vi "Increment File Counter.vi"(8 "error in (no error)":errorcluster, 10 "File Path":path, 11 "Text File Sink in":refnum<class "Text File Sink.lvclass">) -> (0 "error out":errorcluster, 2 "File Path out":path, 3 "Text File Sink out":refnum<class "Text File Sink.lvclass">)   [LabVIEW 2016, in "Stream Log.lvlib" / "Text File Sink.lvclass"]
uses:
  <userlib>/Composed Systems/Stream/Log/Text File Sink/Text File Sink.lvclass
  <userlib>/Composed Systems/Stream/Log/Text File Sink/Text File Sink.lvclass/Text File Sink.ctl
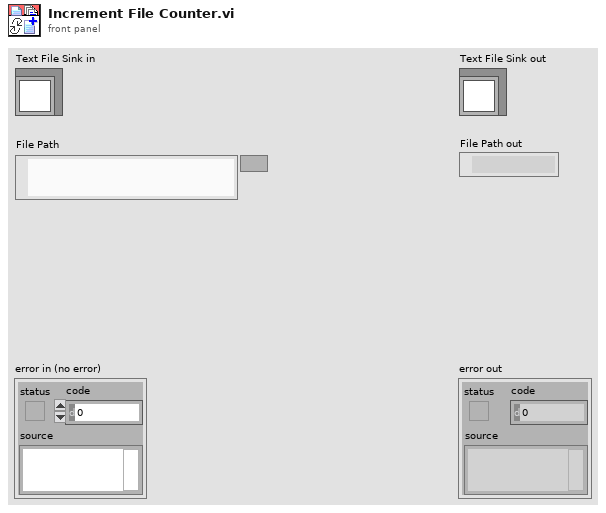
[diagram p1: front panel]
types:
  T1 = typedef "LVDateTimeRec.ctl" = cluster{"fractional second":dbl, "second":i32, "minute":i32, "hour":i32, "day of month":i32, "month":i32, "year":i32, "day of week":i32, "day of year":i32, "DST":i32}
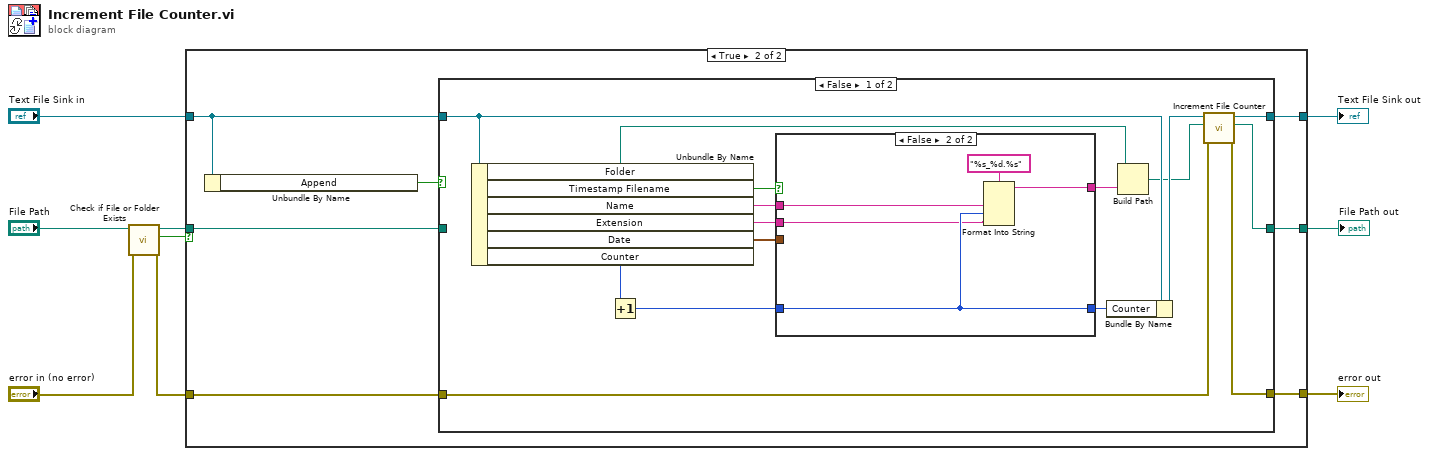
[diagram p0: block diagram]
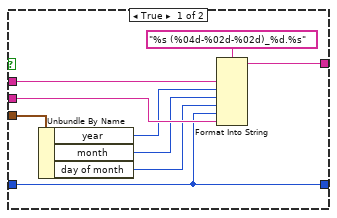
[diagram p3: hidden frame]
diagram:
  n1 = call <vilib>:"Check if File or Folder Exists.vi"("error in (no error)"="error in (no error)", "path"="File Path") -> ("error out"=w2:errorcluster, "file or folder exists?"=w9:bool, "dup path"=w8:path)  [unwired: 7 out]
  n2 = case shown="True" w9 {
    tunnel: w8 -> [w12 w16]
    tunnel: [w12 w17] -> w3
    tunnel: [w11 w15] -> w6
    tunnel: "Text File Sink in" -> [w11 w19]
    tunnel: [w10 w13] -> w1
    tunnel: w2 -> [w10 w14]
    frame False {
    }
    frame True {
      n3 = Unbundle By Name(w19) -> ("Append"=w18:bool)
      n4 = case shown="False" w18 {
        tunnel: [w26 w52] -> w15
        tunnel: w19 -> [w30 w52]
        tunnel: [w25 w51] -> w17
        tunnel: w16 -> [_ w51]
        tunnel: w14 -> [w24 w50]
        tunnel: [w23 w50] -> w13
        frame False {
          n5 = Unbundle By Name(w30) -> ("Folder"=w31:path, "Timestamp Filename"=w20:bool, "Name"=w35:string, "Extension"=w34:string, "Date"=w33:T1, "Counter"=w28:u16)
          n6 = Increment(x=w28) -> (x+1=w29:u16)
          n7 = case shown="False" w20 {
            tunnel: w35 -> [w43 w48]
            tunnel: w34 -> [w42 w45]
            tunnel: w33 -> [w41 _]
            tunnel: [w37 w47] -> w32
            tunnel: w29 -> [w36 w46]
            tunnel: [w36 w46] -> w21
            frame True {
              n8 = Unbundle By Name(w41) -> ("year"=w40:i32, "month"=w39:i32, "day of month"=w38:i32)
              n9 = Format Into String(format string="%s (%04d-%02d-%02d)_%d.%s", w43, w40, w39, w38, w36, w42) -> (resulting string=w37:string)  [unwired: 2 in, 1 out]
            }
            frame False {
              n10 = Format Into String(format string="%s_%d.%s", w48, w46, w45) -> (resulting string=w47:string)  [unwired: 2 in, 1 out]
            }
          }
          n11 = Bundle By Name(cluster=w30, "Counter"=w21) -> (w27:refnum<class "Text File Sink.lvclass">)
          n12 = Build Path(base path=w31, name or relative path=w32) -> (appended path=w22:path)
          n13 = call <userlib>:"Increment File Counter.vi"("error in (no error)"=w24, "File Path"=w22, "Text File Sink in"=w27) -> ("error out"=w23:errorcluster, "File Path out"=w25:path, "Text File Sink out"=w26:refnum<class "Text File Sink.lvclass">)  [unwired: 6 in]
        }
        frame True {
        }
      }
    }
  }
  "error out" <- w1
  "Text File Sink out" <- w6
  "File Path out" <- w3
